vi "Duplicate_DO_WF_4Z.vi"(8 "error in":errorcluster) -> (0 "error out":errorcluster)   [LabVIEW 2025]
uses:
  <vilib>/Waveform/DWDTOps.llb/DWDT Digital Size.vi
  <vilib>/Waveform/DWDTOps.llb/DWDT Append Digital Samples.vi
panel:
  out "Digital waveform 3":digitalwaveform[](graph)
  out "Samples":u32
  in  "Digital waveform 2":digitalwaveform[](graph)
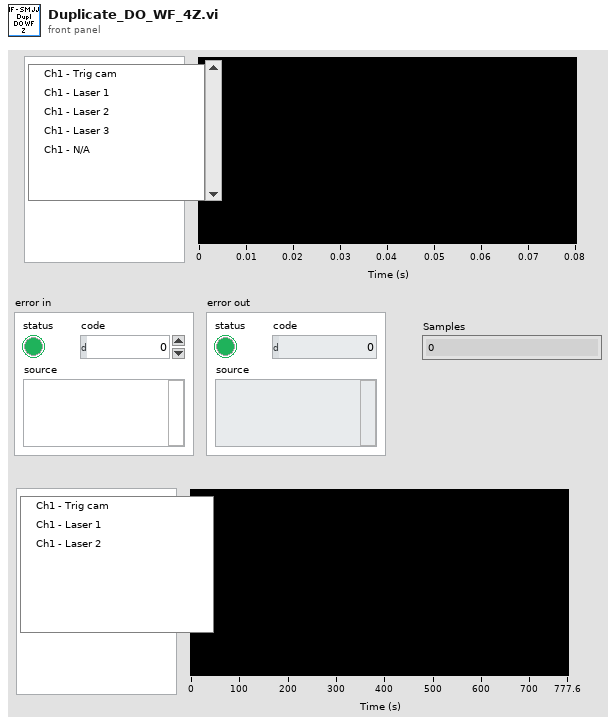
[diagram p1: front panel]
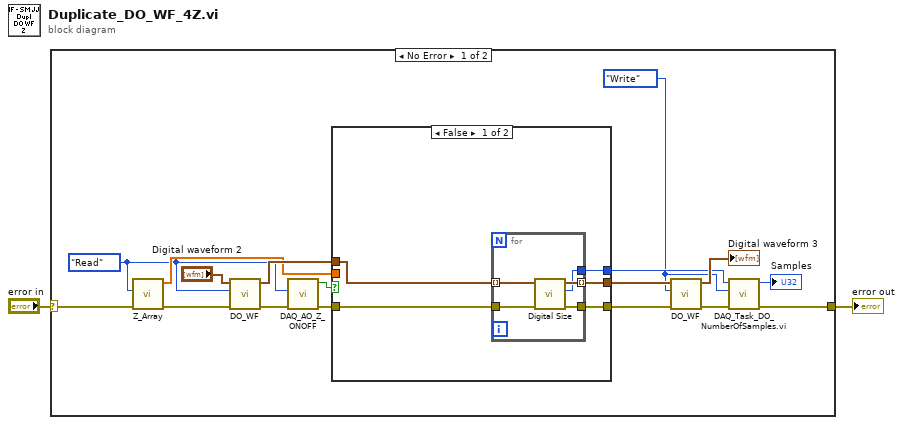
[diagram p0: block diagram]
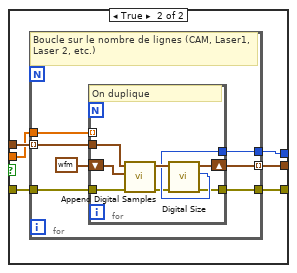
[diagram p2: hidden frame]
diagram:
  n1 = case shown="No Error" "error in" {
    selector: "error in" -> [w15 w51]
    tunnel: [w8 w51] -> w1
    frame No Error {
      w7 = enum16{"Init", "Write", "Read"}."Write" ("Action")
      w5 = enum16{"Init", "Write", "Read"}."Read" ("Action")
      n2 = call "Z_Array.vi"("error in"=w15, "Action"=w5) -> ("error out"=w14:errorcluster, "Z_Array"=w13:dbl[])  [unwired: 8 in]
      n3 = call "DO_WF.vi"("error in"=w14, "Action"=w5, "Digital WF"="Digital waveform 2") -> ("error out"=w6:errorcluster, "Digital WF"=w18:digitalwaveform[])  [unwired: 7 in]
      n4 = call "DAQ_AO_Z_ONOFF.vi"("error in"=w6, "Action"=w5) -> ("error out"=w4:errorcluster, "ON / OFF"=w3:bool)  [unwired: 8 in]
      n5 = case shown="False" w3 {
        tunnel: w4 -> [w23 w35]
        tunnel: w18 -> [w24 w34]
        tunnel: [w22 w33] -> w17
        tunnel: w13 -> [_ w32]
        tunnel: [w21 w31] -> w12
        tunnel: [w20 w30] -> w11
        frame False {
          n6 = for {
            tunnel: w24 -> [w29] mode=indexing
            tunnel: w23 -> [w28]
            tunnel: [w27] -> w22
            tunnel: [w26] -> w21 mode=indexing
            tunnel: [w25] -> w20
            n7 = call-poly <vilib>:"Digital Size.vi"("error in (no error)"=w28, "digital waveform in"=w29) -> ("error out"=w27:errorcluster, "number of samples"=w25:i32, "digital waveform out"=w26:digitalwaveform)  [unwired: 6 in, 1 out]
          }
        }
        frame True {
          n8 = for {
            tunnel: w34 -> [w42] mode=indexing
            tunnel: [w37] -> w31 mode=indexing
            tunnel: w32 -> [w40]
            tunnel: [w36] -> w30
            tunnel: w35 -> [w39]
            tunnel: [w38] -> w33
            # "Boucle sur le nombre de lignes (CAM, Laser1, Laser 2, etc.)"
            n9 = for {
              tunnel: w42 -> [w50]
              shift-right: [w43] -> w37
              shift-left: digitalwaveform {"t0"=timestamp(0 s since 1904-01-01), "dt"=1e-05, "Y"={"transitions"=[], "data"=[]}} ("digital waveform out") -> [w48]
              tunnel: w40 -> [_] mode=indexing
              tunnel: [w46] -> w36
              tunnel: w39 -> [w47]
              tunnel: [w44] -> w38
              # "On duplique"
              n10 = call-poly <vilib>:"Append Digital Samples.vi"("error in (no error)"=w47, "digital waveform B"=w48, "digital waveform A"=w50) -> ("error out"=w45:errorcluster, "digital waveform out"=w49:digitalwaveform)  [unwired: 7 in]
              n11 = call-poly <vilib>:"Digital Size.vi"("error in (no error)"=w45, "digital waveform in"=w49) -> ("error out"=w44:errorcluster, "number of samples"=w46:i32, "digital waveform out"=w43:digitalwaveform)  [unwired: 6 in, 1 out]
            }
          }
        }
      }
      n12 = call "DO_WF.vi"("error in"=w17, "Action"=w7, "Digital WF"=w12) -> ("error out"=w10:errorcluster, "Digital WF"=→"Digital waveform 3":digitalwaveform[])  [unwired: 7 in]
      n13 = call "DAQ_Task_DO_NumberOfSamples.vi.vi"("error in"=w10, "Action"=w7, "Samples"=w11) -> ("error out"=w8:errorcluster, "Samples"=→"Samples":u32)  [unwired: 7 in]
    }
    frame Error {
    }
  }
  "error out" <- w1
